vi "Read CCD Config.vi"(8 "error in (no error)":errorcluster, 11 "CCDCamera in":refnum<class "CCDCamera.lvclass">) -> (0 "error out":errorcluster, 2 "CCD Config":T1, 3 "CCDCamera out":refnum<class "CCDCamera.lvclass">)   [LabVIEW 2018, in "CCDCamera.lvclass"]
uses:
  CCDCamera.lvclass
  CCDCamera.lvclass/CCDCamera.ctl
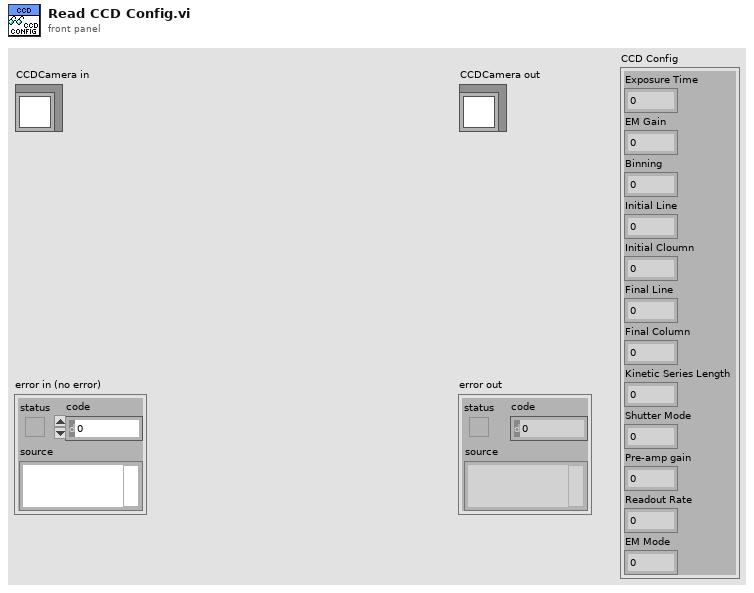
[diagram p1: front panel]
types:
  T1 = cluster{"Exposure Time":sgl, "EM Gain":u16, "Binning":u16, "Initial Line":u16, "Initial Cloumn":u16, "Final Line":u16, "Final Column":u16, "Kinetic Series Length":u32, "Shutter Mode":u8, "Pre-amp gain":u8, "Readout Rate":u8, "EM Mode":u8}
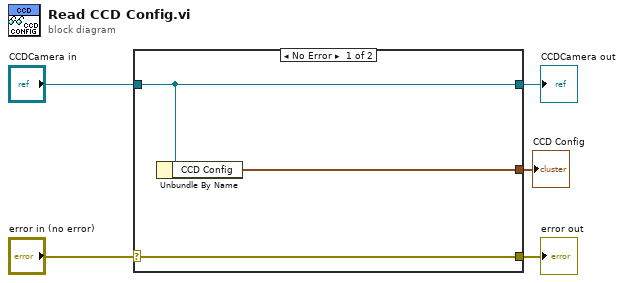
[diagram p0: block diagram]
diagram:
  n1 = case shown="No Error" "error in (no error)" {
    selector: "error in (no error)" -> [w8 w9]
    tunnel: [w8 w9] -> w4
    tunnel: [w7 w10] -> w2
    tunnel: "CCDCamera in" -> [w7 w10]
    tunnel: [w6 _] -> w1
    frame No Error {
      n2 = Unbundle By Name(w7) -> ("CCD Config"=w6:T1)
    }
    frame Error {
    }
  }
  "error out" <- w4
  "CCDCamera out" <- w2
  "CCD Config" <- w1
